vi "Create TDMS_MFP3D.vi"(10 "TDMS File Name":string, 11 "TDMS Output Folder":path) -> (2 "modified path":path, 3 "Refnum out":refnum<k34>)   [LabVIEW 2019]
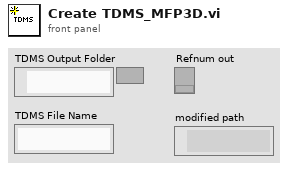
[diagram p1: front panel]
types:
  T1 = enum16{"open", "open or create", "create or replace", "create", "open (read-only)"}
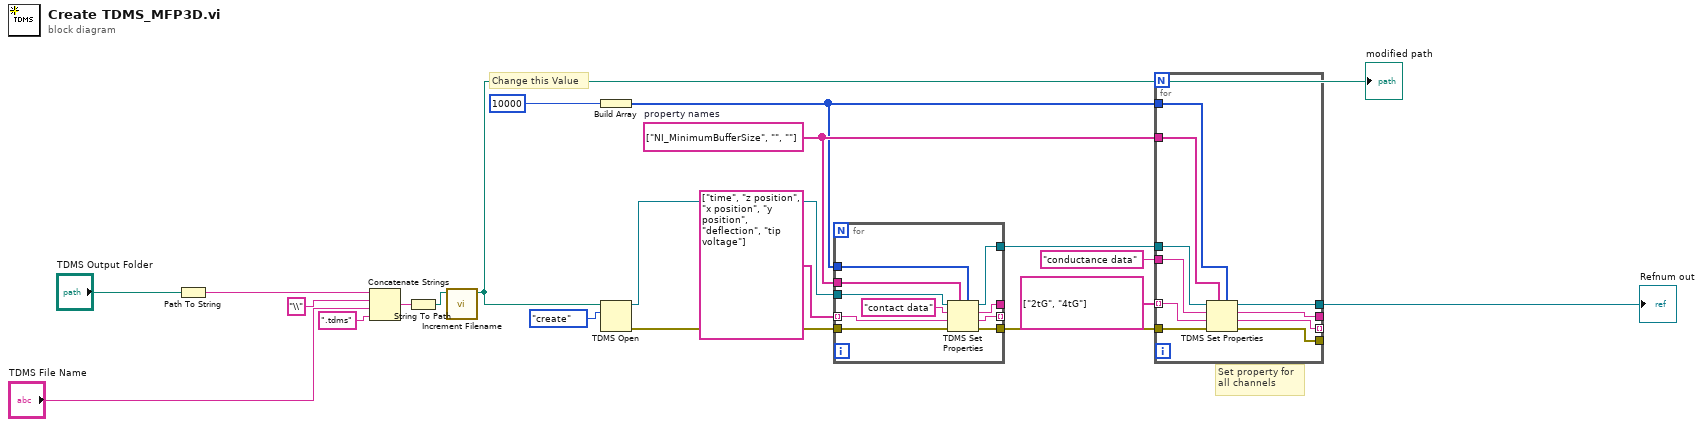
[diagram p0: block diagram]
diagram:
  w7 = string[] ["NI_MinimumBufferSize", "", ""]  # property names
  # "Set property for \nall channels"
  # "Change this Value"
  n1 = Path To String(path="TDMS Output Folder") -> (string=w12:string)
  n2 = Concatenate Strings(w12, "\\" ("name or relative path"), "TDMS File Name", ".tdms" ("name or relative path")) -> (w13:string)
  n3 = String To Path(string=w13) -> (path=w14:path)
  n4 = call <userlib>:"Increment Filename.vi"("Path"=w14) -> ("Modified Path"=w19:path)  [unwired: 9 in, 1 out]
  "modified path" <- w19
  n5 = Build Array(10000) -> (w6:i32[])
  n6 = TDMS Open(10:T1."create" ("operation (0:open)"), 11:w19) -> (0:w3:errorcluster, 3:w11:refnum<k34>)  [unwired: 5 in]
  n7 = for {
    tunnel: [w30] -> w5
    tunnel: [w29] -> w10
    tunnel: w6 -> [w28]
    tunnel: w7 -> [w27]
    tunnel: w11 -> [w26]
    tunnel: w3 -> [w25]
    tunnel: [w24] -> _ mode=indexing
    tunnel: string[] ["time", "z position", "x position", "y position", "deflection", "tip voltage"] -> [w23] mode=indexing
    tunnel: [w22] -> _
    n8 = TDMS Set Properties(5:w28, 7:w27, 8:w25, 9:w23, 10:"contact data", 11:w26) -> (0:w29:errorcluster, 1:w24:string, 2:w22:string, 3:w30:refnum<k34>)
  }
  n9 = for {
    tunnel: [w40] -> w20
    tunnel: [w39] -> _
    tunnel: w6 -> [w38]
    tunnel: w7 -> [w37]
    tunnel: w5 -> [w36]
    tunnel: w10 -> [w35]
    tunnel: [w34] -> _ mode=indexing
    tunnel: string[] ["2tG", "4tG"] -> [w33] mode=indexing
    tunnel: "conductance data" -> [w32]
    tunnel: [w31] -> _
    n10 = TDMS Set Properties(5:w38, 7:w37, 8:w35, 9:w33, 10:w32, 11:w36) -> (0:w39:errorcluster, 1:w34:string, 2:w31:string, 3:w40:refnum<k34>)
  }
  "Refnum out" <- w20
